vi "Get Robot Competition Mode.vi"(11 "DS Occurrence":refnum<k4>) -> (1 "RawControlByte":u8 format="%08b", 2 "Call Context":T1, 3 "Robot Mode":T2)   [LabVIEW 2011]
doc: "<b>Get Competition Mode.vi</b> returns the mode of the current phase of competition, which determines the current restrictions of robot operation that apply. Possible modes include <b>Autonomous Disabled</b>, <b>Autonomous Enabled</b>, <b>Teleop Disabled</b>, and <b>Teleop Enabled</b>.\n\nThis software is licensed. Open the labview\\readme\\WPI Robotics Library Open Source License.txt file for more information."
uses:
  <vilib>/Rock Robotics/WPI/DriverStation/WPI_DriverStationRobotMode.ctl
  <vilib>/Rock Robotics/WPI/DriverStation/WPI_DriverStationDerivedRobotMode.ctl
  <vilib>/Rock Robotics/WPI/DriverStation/WPI_DriverStationCommDataCacheOp.ctl
  signals/Signal.ctl
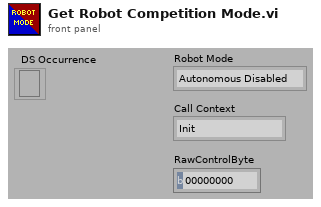
[diagram p1: front panel]
types:
  T1 = typedef "WPI_DriverStationDerivedRobotMode.ctl" = enum16{"Init", "Execute", "Stop"}
  T2 = typedef "WPI_DriverStationRobotMode.ctl" = enum16{"Autonomous Disabled", "Autonomous Enabled", "Teleop Disabled", "Teleop Enabled", "Timeout", "Finish"}
  T3 = typedef "WPI_DriverStationCommDataCacheOp.ctl" = enum16{"Get", "Set", "Init"}
  T4 = typedef "Signal.ctl" = enum16{"SIGFIRE", "SIGSTOPSCRIPT", "SIGSTARTGUN", "SIGSTOPGUN", "SIGDISABLED", "SIGENABLED", "SIGUDPTIMEOUT", "SIGNEWVISION_REMOTE", "SIGNEWVISION_LOCAL", "SIGSHOTFIRED", "SIGDOTRACK", "SIGDONTTRACK"}
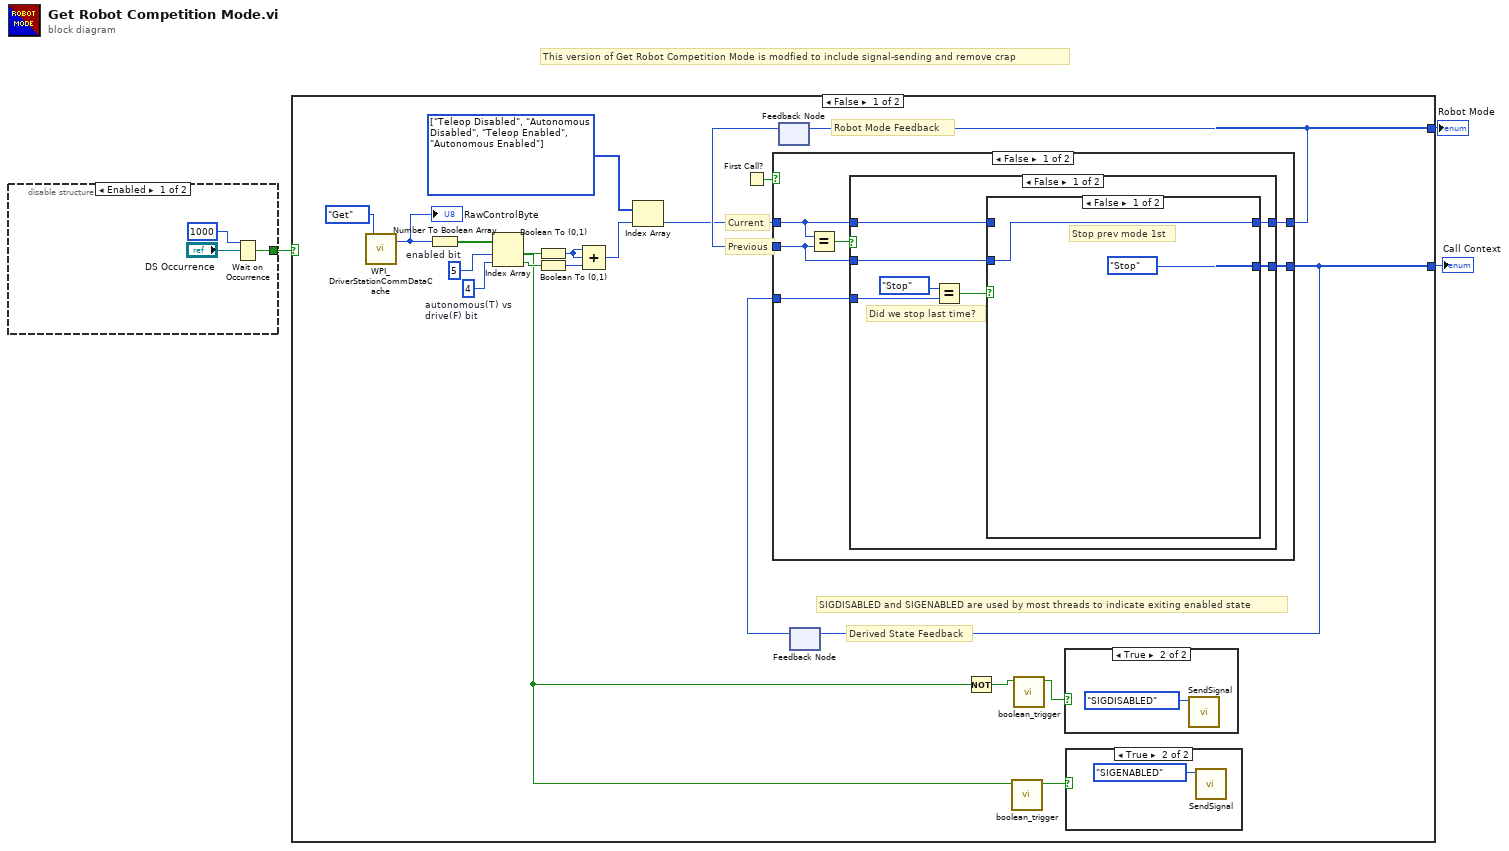
[diagram p0: block diagram]
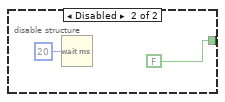
[diagram p2: hidden frame]
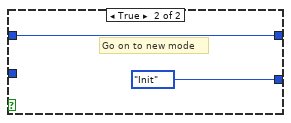
[diagram p5: hidden frame]
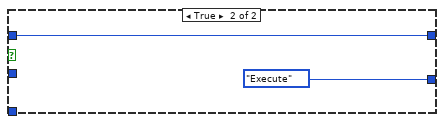
[diagram p6: hidden frame]
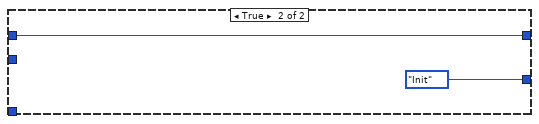
[diagram p7: hidden frame]
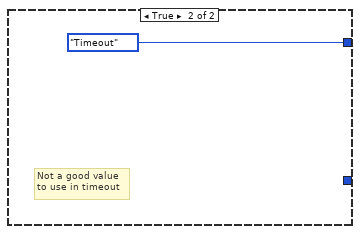
[diagram p8: hidden frame]
diagram:
  # "This version of Get Robot Competition Mode is modfied to include signal-sending and remove crap"
  n1 = disable-structure shown="Enabled" {
    disable-tunnel: [w5 FALSE] -> w1
    frame Enabled {
      n2 = Wait on Occurrence(2:"DS Occurrence", 3:1000 ("ms timeout (-1)")) -> (0:w5:bool)  [unwired: 1 out]
    }
    frame Disabled {
      n3 = Wait (ms)(milliseconds to wait=u32 20) -> ()  [unwired: 1 out]
    }
  }
  n4 = case shown="False" w1 {
    tunnel: [w20 _] -> w3
    tunnel: [w19 WPI_DriverStationRobotMode."Timeout" ("RobotMode")] -> w2
    frame False {
      w18 = T2[] [enum."Teleop Disabled", enum."Autonomous Disabled", enum."Teleop Enabled", enum."Autonomous Enabled"] items=["Autonomous Disabled", "Autonomous Enabled", "Teleop Disabled", "Teleop Enabled", "Timeout", "Finish"]
      w24 = 4  # autonomous(T) vs drive(F) bit
      w25 = 5  # enabled bit
      # "SIGDISABLED and SIGENABLED are used by most threads to indicate exiting enabled state"
      # "Derived State Feedback"
      # "Robot Mode Feedback"
      # "Previous"
      # "Current"
      n5 = call <vilib>:"WPI_DriverStationCommDataCache.vi"("CommDataCacheOp"=WPI_DriverStationCommDataCacheOp."Get") -> ("ControlBit out"=w27:u8)  [unwired: 18 out]
      "RawControlByte" <- w27
      n6 = Number To Boolean Array(number=w27) -> (Boolean array=w26:bool[])
      n7 = Index Array(array=w26, index #1=w25, index #2=w24) -> (element #1=w12:bool, element #2=w15:bool)
      n8 = Boolean To (0,1)(Boolean=w12) -> (0, 1=w17:i16)
      n9 = Boolean To (0,1)(Boolean=w15) -> (0, 1=w16:i16)
      n10 = Compound Arithmetic op=ADD(w17, w17, w16) -> (w14:i16)
      n11 = Index Array(array=w18, index=w14) -> (element=w13:T2)
      n12 = First Call?() -> (First Call?: T/F=w21:bool)
      n13 = feedback #1() -> (w22:T2)  [unwired: 1 out]
      n14 = feedback #2() -> (w23:T1)  [unwired: 1 out]
      n15 = case shown="False" w21 {
        tunnel: [w36 w50] -> w19
        tunnel: [w35 WPI_DriverStationDerivedRobotMode."Init" ("Derived Robot State")] -> w20
        tunnel: w23 -> [w33 _]
        tunnel: w13 -> [w32 w50]
        tunnel: w22 -> [w31 _]
        frame False {
          n16 = Equal?(x=w32, y=w31) -> (x = y?=w34:bool)
          n17 = case shown="False" w34 {
            tunnel: w32 -> [w41 w49]
            tunnel: [w40 w49] -> w36
            tunnel: [w39 WPI_DriverStationDerivedRobotMode."Execute" ("Derived Robot State")] -> w35
            tunnel: w33 -> [w43 _]
            tunnel: w31 -> [w38 _]
            frame False {
              # "Did we stop last time?"
              n18 = Equal?(x=WPI_DriverStationDerivedRobotMode."Stop" ("Derived Robot State"), y=w43) -> (x = y?=w42:bool)
              n19 = case shown="False" w42 {
                tunnel: w41 -> [_ w46]
                tunnel: [w44 w46] -> w40
                tunnel: [WPI_DriverStationDerivedRobotMode."Stop" ("Derived Robot State") WPI_DriverStationDerivedRobotMode."Init" ("Derived Robot State")] -> w39
                tunnel: w38 -> [w44 _]
                frame False {
                  # "Stop prev mode 1st"
                }
                frame True {
                  # "Go on to new mode"
                }
              }
            }
            frame True {
            }
          }
        }
        frame True {
        }
      }
      n20 = feedback-in #1(w19) -> ()
      n21 = feedback-in #2(w20) -> ()
      n22 = Not(x=w12) -> (.not. x?=w9:bool)
      n23 = call "boolean_trigger.vi"("Input"=w12) -> ("Rising Edge"=w11:bool)  [unwired: 10 in]
      n24 = call "boolean_trigger.vi"("Input"=w9) -> ("Rising Edge"=w10:bool)  [unwired: 10 in]
      n25 = case shown="True" w10 {
        frame False {
        }
        frame True {
          n26 = call "SendSignal.vi"("Signal"=Signal."SIGDISABLED") -> ()  [unwired: 11 in]
        }
      }
      n27 = case shown="True" w11 {
        frame False {
        }
        frame True {
          n28 = call "SendSignal.vi"("Signal"=Signal."SIGENABLED") -> ()  [unwired: 11 in]
        }
      }
    }
    frame True {
      # "Not a good value\nto use in timeout"
    }
  }
  "Robot Mode" <- w2
  "Call Context" <- w3
